vi "check for event.vi"(10 "queue index":i32, 11 "event queue in":T2) -> (1 "empty?":bool, 2 "event":T1, 3 "event queue out":T2)   [LabVIEW 2013, in "data bus events.lvlib"]
uses:
  data bus events.lvlib
  event queue.ctl
  event queue element.ctl
  event.ctl
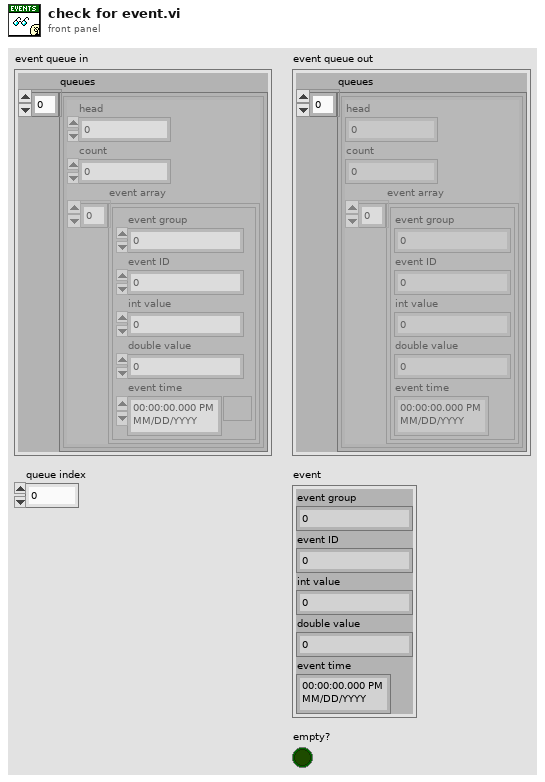
[diagram p1: front panel]
types:
  T1 = typedef "data bus events.lvlib/event.ctl" = cluster{"event group":i64, "event ID":i64, "int value":i64, "double value":dbl, "event time":timestamp}
  T2 = typedef "data bus events.lvlib/event queue.ctl" = cluster{"queues":T3[]}
  T3 = typedef "data bus events.lvlib/event queue element.ctl" = cluster{"head":i32, "count":i32, "event array":T1[]}
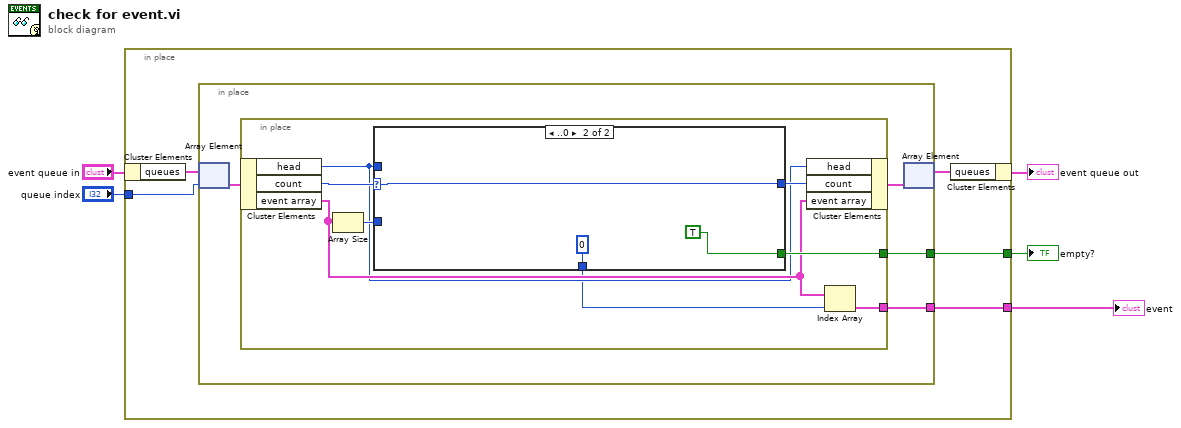
[diagram p0: block diagram]
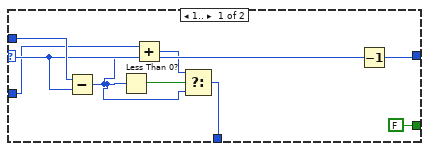
[diagram p2: hidden frame]
diagram:
  n1 = in-place {
    in-place-border: "queue index" -> [w8]
    in-place-border: [w7] -> w2
    in-place-border: [w6] -> w1
    n2 = in-place-cluster #1("event queue in") -> ("queues"=w10:T3[])
    n3 = in-place {
      in-place-border: [w12] -> w7
      in-place-border: [w11] -> w6
      n4 = in-place-array #2(w10, w8) -> (w14:T3)
      n5 = in-place {
        in-place-border: [w21] -> w12
        in-place-border: [w19] -> w11
        n6 = in-place-cluster #3(w14) -> ("head"=w16:i32, "count"=w22:i32, "event array"=w18:T1[])
        n7 = Array Size(array=w18) -> (size(s)=w17:i32)
        n8 = case shown="..0" w22 {
          selector: w22 -> [w28 w33]
          tunnel: w16 -> [w29 _]
          tunnel: [FALSE TRUE] -> w21
          tunnel: [w31 w33] -> w20
          tunnel: w17 -> [w26 _]
          tunnel: [w23 0] -> w15
          frame 1.. {
            n9 = Subtract(x=w29, y=w28) -> (x-y=w24:i32)
            n10 = Less Than 0?(x=w24) -> (x < 0?=w27:bool)
            n11 = Add(x=w26, y=w24) -> (x+y=w25:i32)
            n12 = Select(t=w25, s=w27, f=w24) -> (s? t:f=w23:i32)
            n13 = Decrement(x=w28) -> (x-1=w31:i32)
          }
          frame ..0 {
          }
        }
        n14 = in-place-cluster #3("head"=w16, "count"=w20, "event array"=w18) -> (w13:T3)
        n15 = Index Array(array=w18, index=w15) -> (element=w19:T1)
      }
      n16 = in-place-array #2(w13) -> (w9:T3[])  [unwired: 1 out]
    }
    n17 = in-place-cluster #1("queues"=w9) -> (→"event queue out":T2)
  }
  "empty?" <- w2
  "event" <- w1
